vi "GMLAN ReportProgrammedState.vi"(8 "error in (no error)":errorcluster, 11 "diag ref in":T2={"Diag CAN Handle"=0, "Transport Protocol"=enum."ISO TP - Normal Mode", "Receive Address Extension"=0, "Transmit Address Extension"=0, "Receive CAN Id"=0, "Transmit CAN Id"=0, "Log Frames ?"=FALSE, "My TP Address"=0, "Other TP Address"=0, "T1"=0, "T2"=0, "T3"=0, "T4"=0, "Tx SN"=0, "Block Size"=0, "Rx SN"=0, "VW TP Initialized?"=FALSE, "Tx block no"=0, "baud rate"=0, "Interface"="", "Channel Diag CAN Handle"=0, "UDP Connection ID"=refnum, "TCP Connection ID"=refnum, "Target IP Addr"=0, "Source Address"=0, "Target Address"=0, "Send Header NACK?"=FALSE, "DLL Handle"=0, "NAD"=0, "Time Stamp read first"=0.0, "Time Stamp read last"=0.0, "Time Stamp write first"=0.0, "Time Stamp write last"=0.0, "Time Stamp write"=0.0, "Time Stamp read"=0.0, " I/O Mode"=0, "FD Baudrate"=0, "TX_DL"=8, "RX_DL"=8, "DoIP Protocol Version"=1, " Selected I/O Mode"=0, "TesterPresent Counter"=0, "TesterPresent Limit"=0, "TesterPresent Tick[ms]"=10, "TesterPresent RequireResponse?"=FALSE, "TesterPresent Stored Ref?"=FALSE, "TesterPresent Message"=[], "TesterPresent Task Handle"=0, "TesterPresent Semaphore"=refnum, "Response Plausibility Check"=1, "Default Version?"=TRUE, "Diagostic Globals"={"Timeout FC (Bs)"=250, "Timeout CF (Cr)"=250, "Timeout Diag Command"=1000, "Receive Block Size (BS)"=0, "Wait Time CF (STmin)"=5, "Max Waits (N_WFTmax)"=10, "Waits to Send (N_WAIT)"=0, "Time between Waits (TW)"=25, "Fill CAN Frames?"=TRUE, "Fill Byte"=255, "Invalid Response as Error?"=FALSE, "Max RspPending Count"=5, "VWTP Command Timeout"=50, "Transport Protocol"=enum."Diagnostics on IP", "Diag CAN Handle"=0, "DLL Handle"=0, "Timeout RspPending"=1000}, "Session-based Properties?"=FALSE} {"Diagostic Globals"."Fill Byte" format="%x"; "TesterPresent Message" format="%.0x"; "Selected I/O Mode" items=["CAN", "CAN FD", "CAN FD+BRS", "ECU Determined"]; "DoIP Protocol Version" items=["2010"=1, "2012"=2]; "RX_DL" items=["8"=8, "12"=12, "16"=16, "20"=20, "24"=24, "32"=32, "48"=48, "64"=64]; "TX_DL" items=["8"=8, "12"=12, "16"=16, "20"=20, "24"=24, "32"=32, "48"=48, "64"=64]; "I/O Mode" items=["CAN", "CAN FD", "CAN FD+BRS", "Not yet determined"]}) -> (0 "error out":errorcluster, 1 "success?":bool, 2 "programmedState":T1 items=["fully programmed"=0, "no op s/w or cal data"=1, "op s/w present, cal data missing"=2, "s/w present, default or no start cal present"=3, "General Memory Fault"=80, "RAM Memory Fault"=81, "NVRAM Memory Fault"=82, "Boot Memory Failure"=83, "Flash Memory Failure"=84, "Flash Memory Failure"=85], 3 "diag ref out":T2={"Diag CAN Handle"=0, "Transport Protocol"=enum."ISO TP - Normal Mode", "Receive Address Extension"=0, "Transmit Address Extension"=0, "Receive CAN Id"=0, "Transmit CAN Id"=0, "Log Frames ?"=FALSE, "My TP Address"=0, "Other TP Address"=0, "T1"=0, "T2"=0, "T3"=0, "T4"=0, "Tx SN"=0, "Block Size"=0, "Rx SN"=0, "VW TP Initialized?"=FALSE, "Tx block no"=0, "baud rate"=0, "Interface"="", "Channel Diag CAN Handle"=0, "UDP Connection ID"=refnum, "TCP Connection ID"=refnum, "Target IP Addr"=0, "Source Address"=0, "Target Address"=0, "Send Header NACK?"=FALSE, "DLL Handle"=0, "NAD"=0, "Time Stamp read first"=0.0, "Time Stamp read last"=0.0, "Time Stamp write first"=0.0, "Time Stamp write last"=0.0, "Time Stamp write"=0.0, "Time Stamp read"=0.0, " I/O Mode"=0, "FD Baudrate"=0, "TX_DL"=8, "RX_DL"=8, "DoIP Protocol Version"=1, " Selected I/O Mode"=0, "TesterPresent Counter"=0, "TesterPresent Limit"=0, "TesterPresent Tick[ms]"=10, "TesterPresent RequireResponse?"=FALSE, "TesterPresent Stored Ref?"=FALSE, "TesterPresent Message"=[], "TesterPresent Task Handle"=0, "TesterPresent Semaphore"=refnum, "Response Plausibility Check"=1, "Default Version?"=TRUE, "Diagostic Globals"={"Timeout FC (Bs)"=250, "Timeout CF (Cr)"=250, "Timeout Diag Command"=1000, "Receive Block Size (BS)"=0, "Wait Time CF (STmin)"=5, "Max Waits (N_WFTmax)"=10, "Waits to Send (N_WAIT)"=0, "Time between Waits (TW)"=25, "Fill CAN Frames?"=TRUE, "Fill Byte"=255, "Invalid Response as Error?"=FALSE, "Max RspPending Count"=5, "VWTP Command Timeout"=50, "Transport Protocol"=enum."Diagnostics on IP", "Diag CAN Handle"=0, "DLL Handle"=0, "Timeout RspPending"=1000}, "Session-based Properties?"=FALSE} {"Diagostic Globals"."Fill Byte" format="%x"; "TesterPresent Message" format="%.0x"; "Selected I/O Mode" items=["CAN", "CAN FD", "CAN FD+BRS", "ECU Determined"]; "DoIP Protocol Version" items=["2010"=1, "2012"=2]; "RX_DL" items=["8"=8, "12"=12, "16"=16, "20"=20, "24"=24, "32"=32, "48"=48, "64"=64]; "TX_DL" items=["8"=8, "12"=12, "16"=16, "20"=20, "24"=24, "32"=32, "48"=48, "64"=64]; "I/O Mode" items=["CAN", "CAN FD", "CAN FD+BRS", "Not yet determined"]})   [LabVIEW 2019, in "GMLAN.lvlib"]
uses:
  GMLAN.lvlib
  <vilib>/Automotive Diagnostic Command Set/Diagnostic Transport.llb/Diag Reference.ctl
  <vilib>/Automotive Diagnostic Command Set/Diagnostic Transport.llb/Transport Protocol Selector.ctl
  <vilib>/Automotive Diagnostic Command Set/Diagnostic Transport.llb/DoIP Protocol Version.ctl
  <vilib>/Automotive Diagnostic Command Set/Diagnostic Transport.llb/Diag Globals.ctl
  _Types/ReportProgrammedState_programmedState.ctl
  <vilib>/Automotive Diagnostic Command Set/Diagnostic Transport.llb/Diagnostic Service Send.vi
  <vilib>/Automotive Diagnostic Command Set/Diagnostic Transport.llb/Diagnostic Response Recv.vi
  <vilib>/Automotive Diagnostic Command Set/Diagnostic Transport.llb/ISOTP Transmit.vi
  <vilib>/Automotive Diagnostic Command Set/Diagnostic Transport.llb/ISOTP7 Transmit.vi
  <vilib>/Automotive Diagnostic Command Set/Diagnostic Transport.llb/DoIP Transmit.vi
  <vilib>/Automotive Diagnostic Command Set/Diagnostic Transport.llb/LIN ISOTP Transmit.vi
  <vilib>/Automotive Diagnostic Command Set/Diagnostic Transport.llb/Diagnostic Service Recv.vi
  <vilib>/Automotive Diagnostic Command Set/Diagnostic Transport.llb/ISOTP Send FF.vi
  <vilib>/Automotive Diagnostic Command Set/Diagnostic Transport.llb/ISOTP Send CFs.vi
  <vilib>/Automotive Diagnostic Command Set/Diagnostic Transport.llb/ISOTP Send Frame.vi
  <vilib>/Automotive Diagnostic Command Set/Diagnostic Transport.llb/ISOTP7 Send FF.vi
  <vilib>/Automotive Diagnostic Command Set/Diagnostic Transport.llb/ISOTP7 Send CFs.vi
  <vilib>/Automotive Diagnostic Command Set/Diagnostic Transport.llb/ISOTP7 Send Frame.vi
  <vilib>/Automotive Diagnostic Command Set/Diagnostic Transport.llb/DoIP TCP Msg Send.vi
  <vilib>/Automotive Diagnostic Command Set/Diagnostic Transport.llb/DoIP TCP Msg Recv.vi
  <vilib>/Automotive Diagnostic Command Set/Diagnostic Transport.llb/DoIP Check Addresses.vi
  <vilib>/Automotive Diagnostic Command Set/Diagnostic Transport.llb/DoIP Check ACK Code.vi
  <vilib>/Automotive Diagnostic Command Set/Diagnostic Transport.llb/ISOTP Receive.vi
  <vilib>/Automotive Diagnostic Command Set/Diagnostic Transport.llb/ISOTP7 Receive.vi
  <vilib>/Automotive Diagnostic Command Set/Diagnostic Transport.llb/DoIP Receive.vi
  <vilib>/Automotive Diagnostic Command Set/Diagnostic Transport.llb/LIN ISOTP Receive.vi
  <vilib>/Automotive Diagnostic Command Set/Diagnostic Transport.llb/Diag Get Globals.vi
  <vilib>/Automotive Diagnostic Command Set/Diagnostic Transport.llb/ISOTP Recv FC.vi
  <vilib>/Automotive Diagnostic Command Set/Diagnostic Transport.llb/ISOTP Send CF.vi
  <vilib>/Automotive Diagnostic Command Set/Diagnostic Transport.llb/Diag Fill Frame.vi
  <vilib>/Automotive Diagnostic Command Set/Diagnostic Transport.llb/ISOTP Calc Send Params.vi
  <vilib>/Automotive Diagnostic Command Set/Diagnostic Transport.llb/ISOTP7 Recv FC.vi
  <vilib>/Automotive Diagnostic Command Set/Diagnostic Transport.llb/ISOTP7 Send CF.vi
  <vilib>/Automotive Diagnostic Command Set/Diagnostic Transport.llb/DoIP Add Addresses.vi
  <vilib>/Automotive Diagnostic Command Set/Diagnostic Transport.llb/DoIP TCP Send.vi
  <vilib>/Automotive Diagnostic Command Set/Diagnostic Transport.llb/DoIP TCP Recv.vi
  <vilib>/Automotive Diagnostic Command Set/Diagnostic Transport.llb/DoIP Add Header.vi
  <vilib>/Automotive Diagnostic Command Set/Diagnostic Transport.llb/ISOTP Recv Frame.vi
  <vilib>/Automotive Diagnostic Command Set/Diagnostic Transport.llb/ISOTP Recv CFs.vi
  <vilib>/Automotive Diagnostic Command Set/Diagnostic Transport.llb/ISOTP7 Recv Frame.vi
  <vilib>/Automotive Diagnostic Command Set/Diagnostic Transport.llb/ISOTP7 Recv CFs.vi
  <vilib>/Automotive Diagnostic Command Set/Diagnostic Transport.llb/DoIP Send Alive.vi
  <vilib>/Automotive Diagnostic Command Set/Diagnostic Transport.llb/DoIP Check Error.vi
  <vilib>/Automotive Diagnostic Command Set/Diagnostic Transport.llb/ISOTP Check Redo.vi
  <vilib>/Automotive Diagnostic Command Set/Diagnostic Transport.llb/ISOTP Recv Block.vi
  <vilib>/Automotive Diagnostic Command Set/Diagnostic Transport.llb/ISOTP7 Recv Block.vi
  <vilib>/Utility/error.llb/Clear Errors.vi
  <vilib>/Automotive Diagnostic Command Set/Diagnostic Transport.llb/ISOTP Send FC.vi
  <vilib>/Automotive Diagnostic Command Set/Diagnostic Transport.llb/ISOTP Add CF.vi
  <vilib>/Automotive Diagnostic Command Set/Diagnostic Transport.llb/ISOTP7 Send FC.vi
  <vilib>/Automotive Diagnostic Command Set/Diagnostic Transport.llb/ISOTP7 Add CF.vi
  <vilib>/Automotive Diagnostic Command Set/Diagnostic Transport.llb/Diag Globals.vi
  <vilib>/Automotive Diagnostic Command Set/Diagnostic Transport.llb/CAN Send Frame Check Queue.vi
  <vilib>/Automotive Diagnostic Command Set/Diagnostic Transport.llb/Diag CAN get timestamp.vi
  <vilib>/Automotive Diagnostic Command Set/Diagnostic Transport.llb/Diag CAN read.vi
  <vilib>/Automotive Diagnostic Command Set/Diagnostic Transport.llb/ISOTP Calc Actual IO Mode.vi
  <vilib>/Automotive Diagnostic Command Set/Diagnostic Transport.llb/ISOTP Get FC Data.vi
  <vilib>/Automotive Diagnostic Command Set/Diagnostic Transport.llb/VWTP Write.vi
  <vilib>/Automotive Diagnostic Command Set/Diagnostic Transport.llb/DoIP Analyze Header.vi
  <vilib>/Automotive Diagnostic Command Set/Diagnostic Transport.llb/Diag CAN status.vi
  <vilib>/Automotive Diagnostic Command Set/Diagnostic Transport.llb/VWTP Read.vi
  <vilib>/Automotive Diagnostic Command Set/Diagnostic Transport.llb/Apply Diagnostic Error.vi
  <vilib>/addons/Automotive Diagnostic Command Set/NI_Automotive Diagnostic Command Set.lvlib
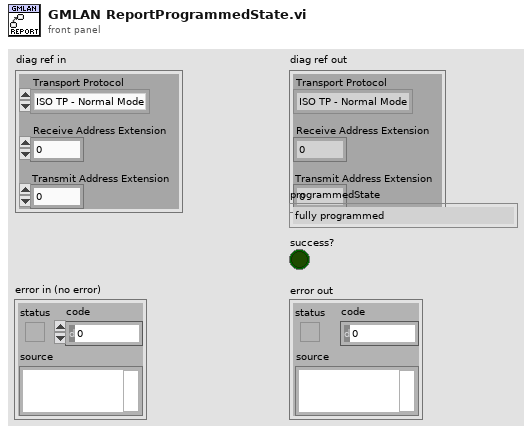
[diagram p1: front panel]
types:
  T1 = typedef "GMLAN.lvlib/ReportProgrammedState_programmedState.ctl" = u8
  T2 = typedef "NI_Automotive Diagnostic Command Set.lvlib/Diag Reference.ctl" = cluster{"Diag CAN Handle":u32, "Transport Protocol":T3, "Receive Address Extension":u8, "Transmit Address Extension":u8, "Receive CAN Id":u32, "Transmit CAN Id":u32, "Log Frames ?":bool, "My TP Address":u8, "Other TP Address":u8, "T1":u16, "T2":u16, "T3":u16, "T4":u16, "Tx SN":u8, "Block Size":u8, "Rx SN":u8, "VW TP Initialized?":bool, "Tx block no":u8, "baud rate":u64, "Interface":string, "Channel Diag CAN Handle":u32, "UDP Connection ID":refnum<k16>, "TCP Connection ID":refnum<k5>, "Target IP Addr":u32, "Source Address":u16, "Target Address":u16, "Send Header NACK?":bool, "DLL Handle":u32, "NAD":u8, "Time Stamp read first":dbl, "Time Stamp read last":dbl, "Time Stamp write first":dbl, "Time Stamp write last":dbl, "Time Stamp write":dbl, "Time Stamp read":dbl, " I/O Mode":u32, "FD Baudrate":u64, "TX_DL":u16, "RX_DL":u16, "DoIP Protocol Version":T4, " Selected I/O Mode":u32, "TesterPresent Counter":u32, "TesterPresent Limit":u32, "TesterPresent Tick[ms]":i32, "TesterPresent RequireResponse?":bool, "TesterPresent Stored Ref?":bool, "TesterPresent Message":u8[], "TesterPresent Task Handle":i32, "TesterPresent Semaphore":T5, "Response Plausibility Check":u32, "Default Version?":bool, "Diagostic Globals":T6, "Session-based Properties?":bool}
  T3 = typedef "NI_Automotive Diagnostic Command Set.lvlib/Transport Protocol Selector.ctl" = enum16{"ISO TP - Normal Mode", "ISO TP - Mixed Mode", "VW TP 2.0", "Diagnostics on IP", "ISO TP LIN"}
  T4 = typedef "NI_Automotive Diagnostic Command Set.lvlib/DoIP Protocol Version.ctl" = u8
  T5 = typedef "Semaphore RefNum" = refnum<k1>
  T6 = typedef "NI_Automotive Diagnostic Command Set.lvlib/Diag Globals.ctl" = cluster{"Timeout FC (Bs)":u32, "Timeout CF (Cr)":u32, "Timeout Diag Command":u32, "Receive Block Size (BS)":u8, "Wait Time CF (STmin)":u8, "Max Waits (N_WFTmax)":u8, "Waits to Send (N_WAIT)":i32, "Time between Waits (TW)":u32, "Fill CAN Frames?":bool, "Fill Byte":u32, "Invalid Response as Error?":bool, "Max RspPending Count":u32, "VWTP Command Timeout":u32, "Transport Protocol":T3, "Diag CAN Handle":u32, "DLL Handle":u32, "Timeout RspPending":u32}
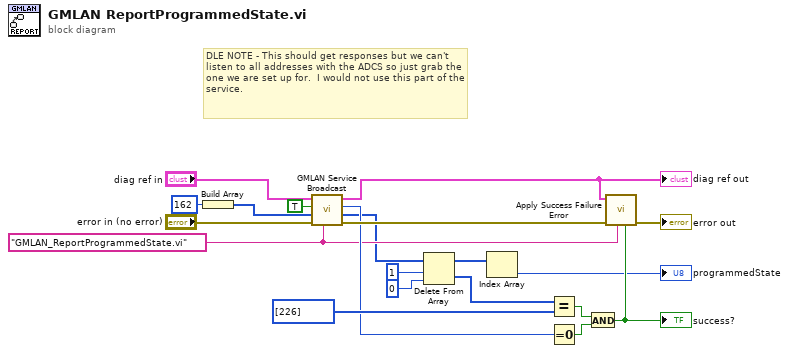
[diagram p0: block diagram]
diagram:
  w8 = "GMLAN_ReportProgrammedState.vi" ("error source")
  # "DLE NOTE - This should get responses but we can't listen to all addresses with the ADCS so just grab the one we are set up for.  I would not use this part of the service."
  n1 = Build Array(u8 162) -> (w17:u8[])
  n2 = call "GMLAN Service Broadcast.vi"("error source"=w8, "error in (no error)"="error in (no error)", "data in"=w17, "require response?"=TRUE, "diag ref in"="diag ref in") -> ("error out"=w10:errorcluster, "data out"=w5:u8[], "error code"=w9:u8, "diag ref out"=w1:T2)  [unwired: 3 in]
  "diag ref out" <- w1
  n3 = Delete From Array(array=w5, length=1, index=0) -> (deleted portion=w4:u8[], array with subset deleted=w3:u8[])
  n4 = Index Array(array=w3) -> (element=→"programmedState":u8)  [unwired: 1 in]
  n5 = Equal?(x=w4, y=u8[] [226]) -> (x = y?=w14:bool)
  n6 = Equal To 0?(x=w9) -> (x = 0?=w13:bool)
  n7 = And(x=w14, y=w13) -> (x .and. y?=w12:bool)
  "success?" <- w12
  n8 = call <vilib>:"Apply Success Failure Error.vi"("success code"=w12, "error source"=w8, "error in (no error)"=w10, "Diag Reference"=w1) -> ("error out"=→"error out":errorcluster)  [unwired: 7 out]
